vi "EnFlo_Lab_Temp_Control.vi"() -> ()   [LabVIEW 2010]
uses:
  ADAM Client/Sub VIs/ADAM Controls/Update_scan_value.ctl
panel:
  out "Total Delta Q":dbl
  out "Q output change from A Tunnel":dbl
  out "Desired Temp":dbl
  out "New Q":dbl
  out "Chiller water temp change OK?":bool
  out "Desired Chilled water temp":dbl
  out "Delta T Chiller":dbl
  out "Delta Q":dbl
  out "Temperature Error":dbl
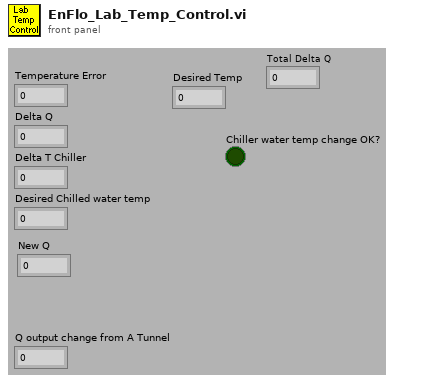
[diagram p1: front panel]
types:
  T1 = typedef "Update_scan_value.ctl" = cluster{"Channel Name":string, "New Value":dbl}
  T2 = enum16{"Append to Global", "Read Global then Clear"}
  T3 = typedef "Ch_description_ADAM.ctl" = cluster{"Ch Name":string, "Type":T4, "Function":T5, "Ch State":T6, "Calibration type":T7, "A":dbl, "B":dbl, "C":dbl, "D":dbl, "Comments":string, "Address":T8, "String":string, "Duty":u16}
  T4 = typedef "Module_type_ADAM.ctl" = enum16{"4011", "4012", "4013", "4014", "4016", "4017", "4018", "4021", "4050", "4052", "4053", "4060", "4080", "5000", "5017", "5018", "5024", "5051", "5056", "5060", "6060", "Tracker", "WEST", "GILL", "JEM", "VICI", "Vaisala", "DRUCK", "Run VI Named:", "IR2100", "PPT", "Comparator", "VIRTUAL", "Hold Value", "Read A", "Read Ch", "Coded", "Client Info", "Web Client", "X10", "Test"}
  T5 = typedef "Function_ADAM.ctl" = enum16{"Analogue Input", "Digital Input", "Event counter", "Event rate", "Analogue Output", "Digital Output", "Relay Output"}
  T6 = typedef "Channel_State.ctl" = enum16{"On", "Off", "Always On", "Always Off"}
  T7 = typedef "Calib_type_ADAM.ctl" = enum16{"Raw", "Bx + A", "Cx^2 + Bx + A", "Dx^3 + Cx^2 + Bx + A", "In Band", "Hi-Tec Q", "Hi-Tec M_dot", "Text"}
  T8 = typedef "Address.ctl" = cluster{"Main":i32, "Ch.":i32, "Sub":i32, "Port Name":string}
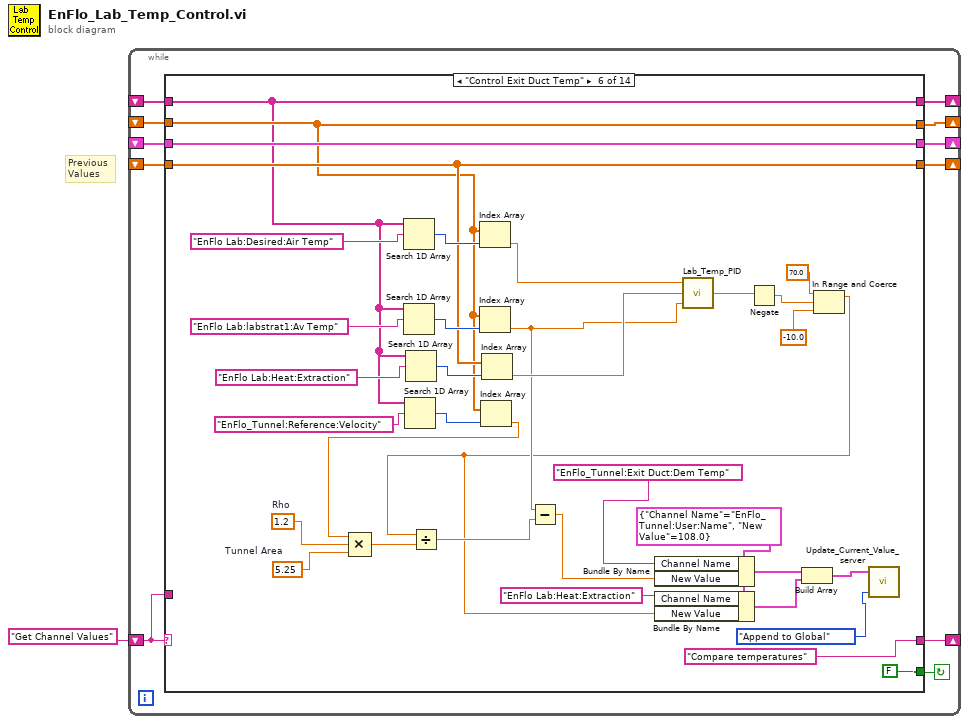
[diagram p0: block diagram]
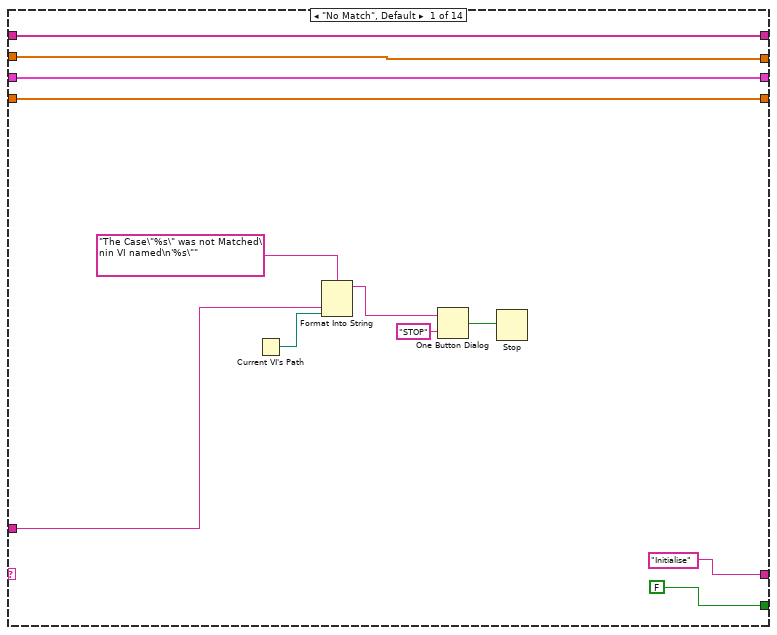
[diagram p2: hidden frame]
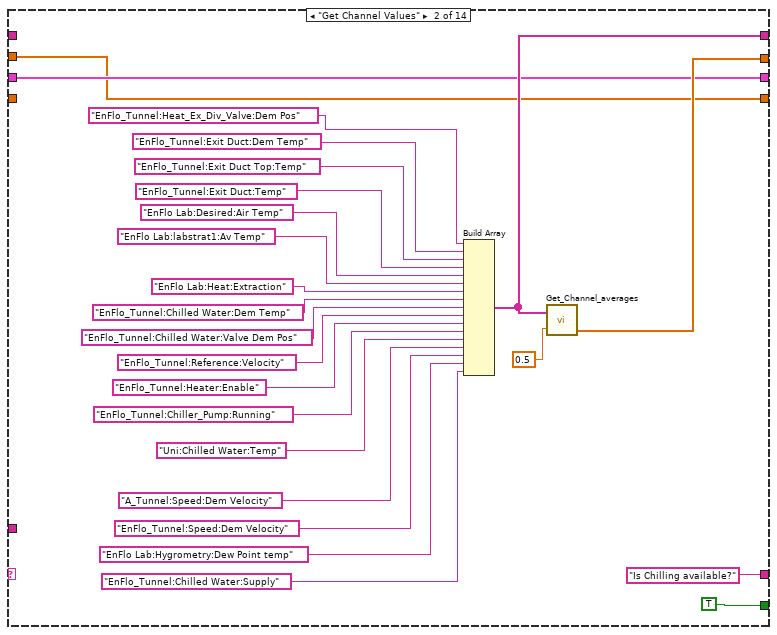
[diagram p3: hidden frame]
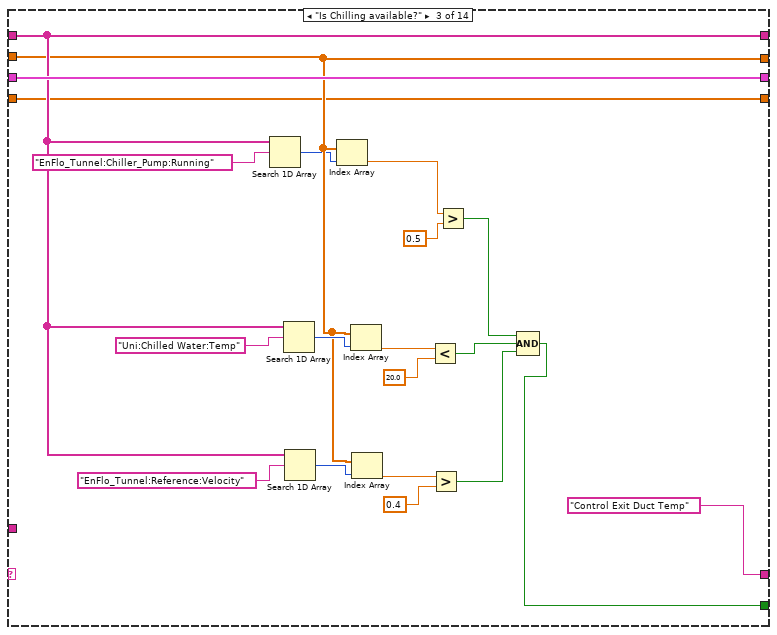
[diagram p4: hidden frame]
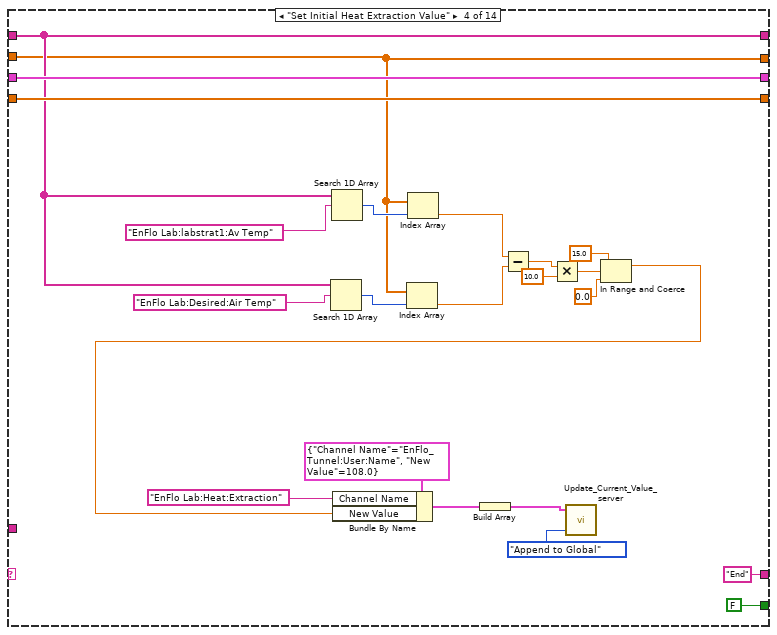
[diagram p5: hidden frame]
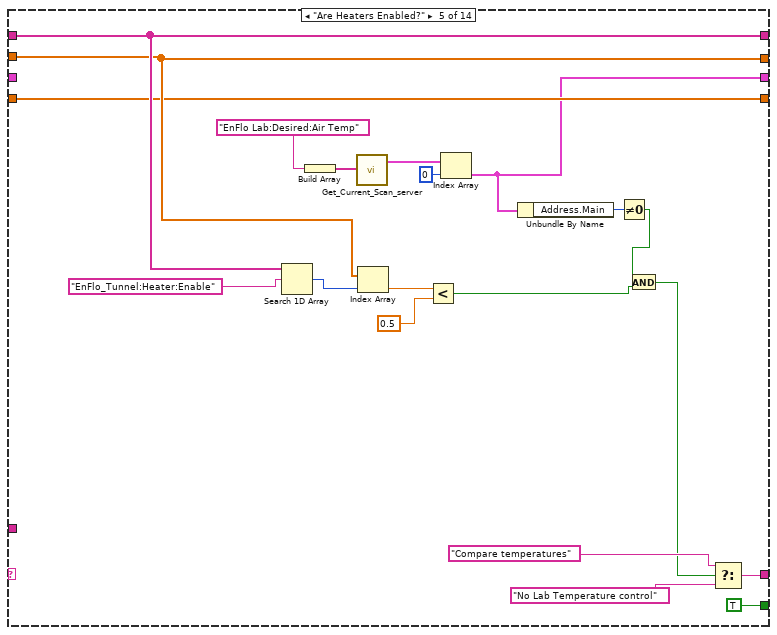
[diagram p6: hidden frame]
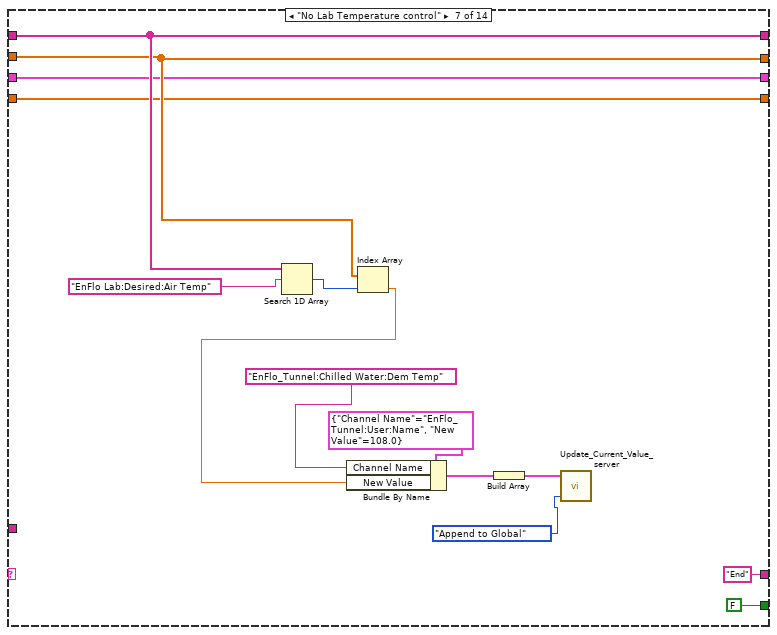
[diagram p7: hidden frame]
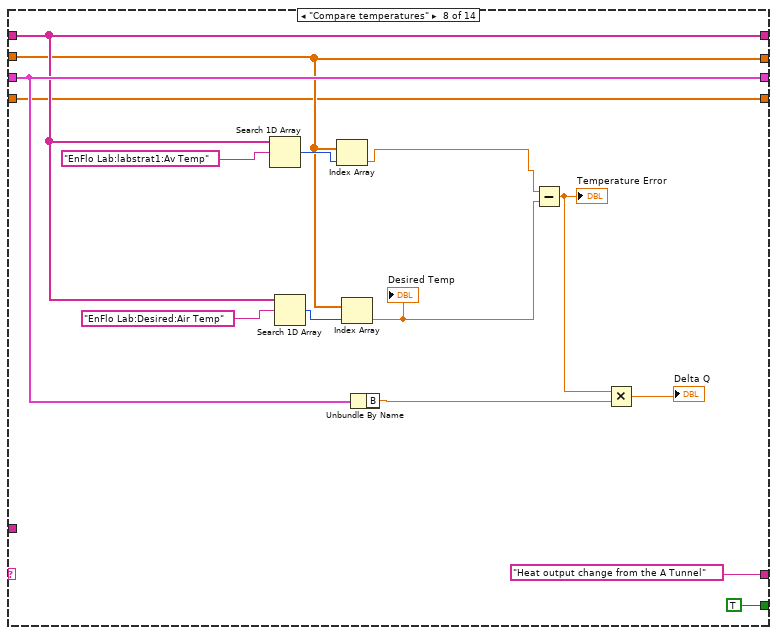
[diagram p8: hidden frame]
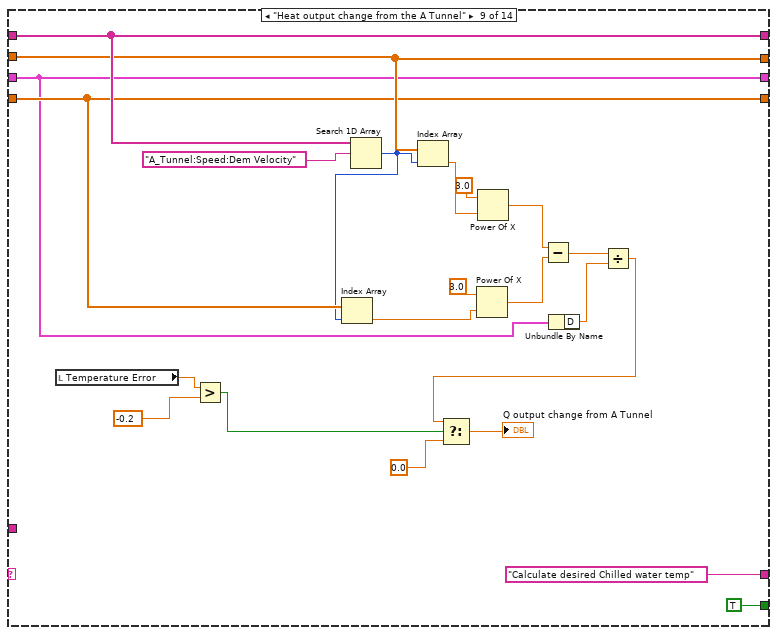
[diagram p9: hidden frame]
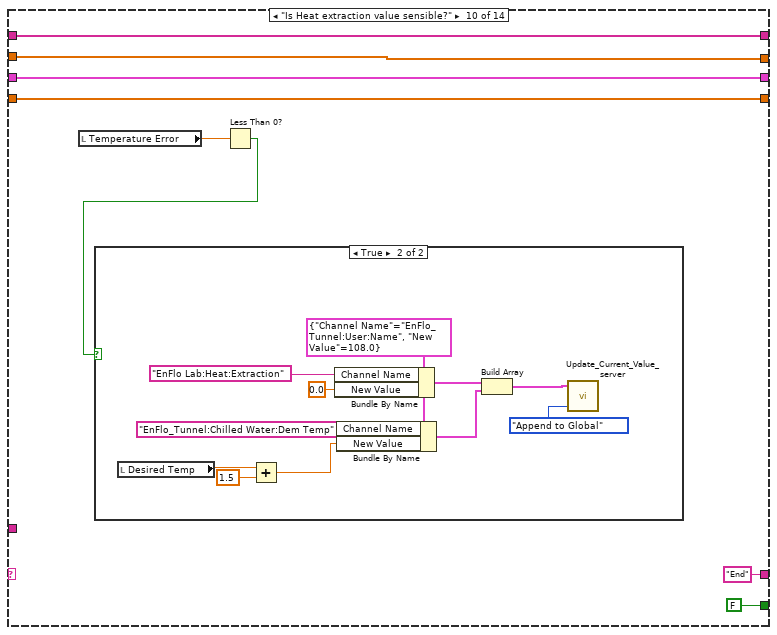
[diagram p10: hidden frame]
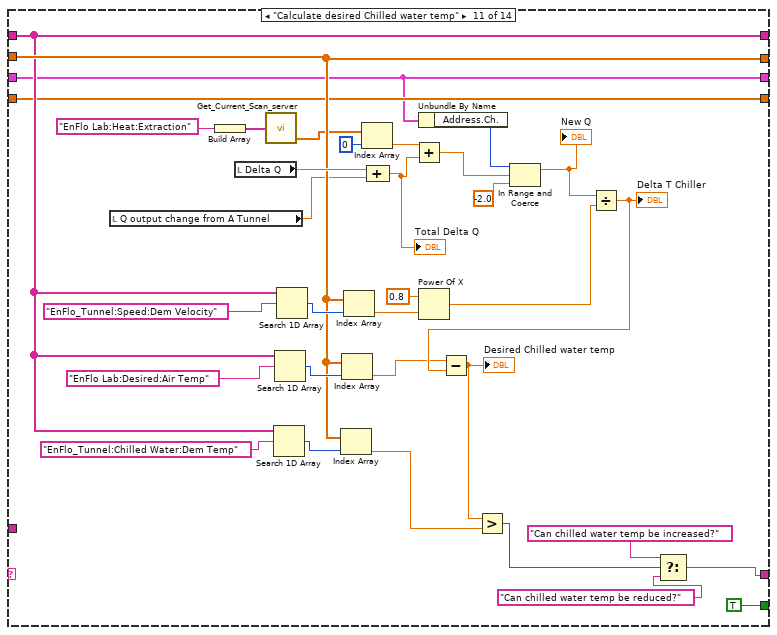
[diagram p12: hidden frame]
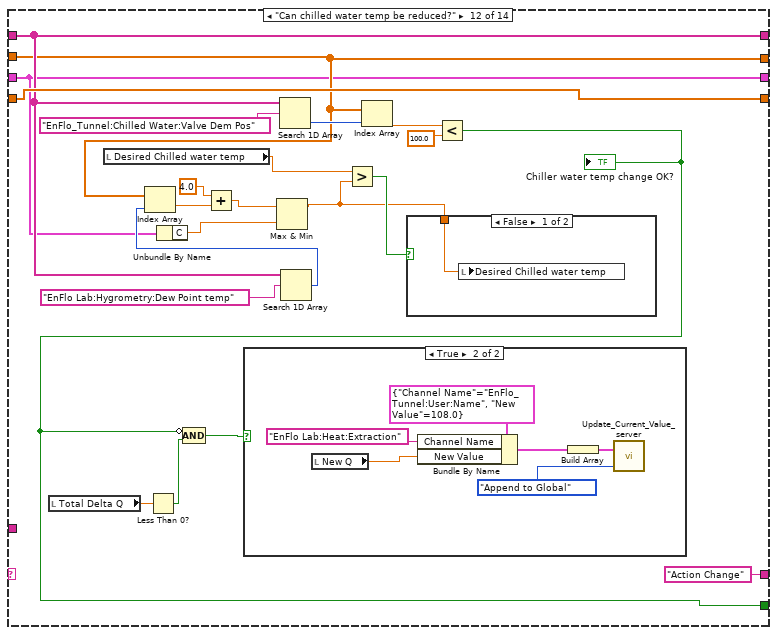
[diagram p13: hidden frame]
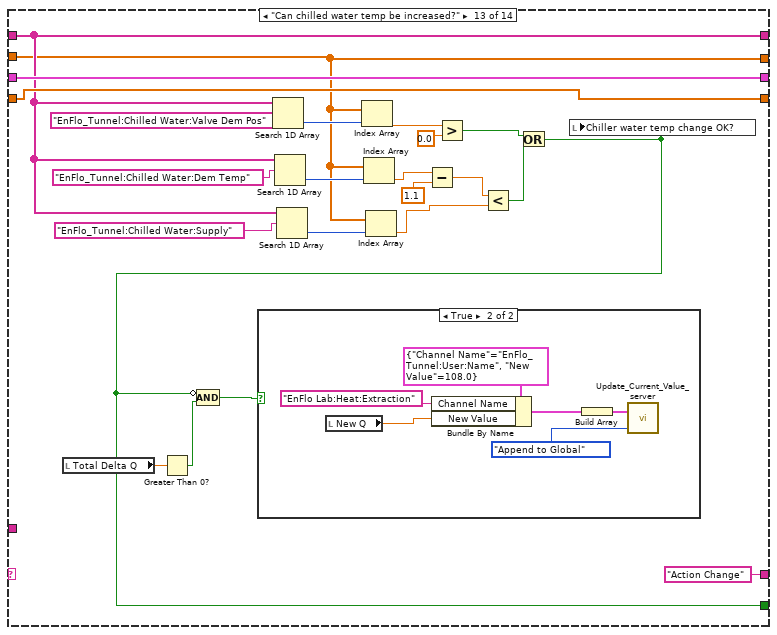
[diagram p16: hidden frame]
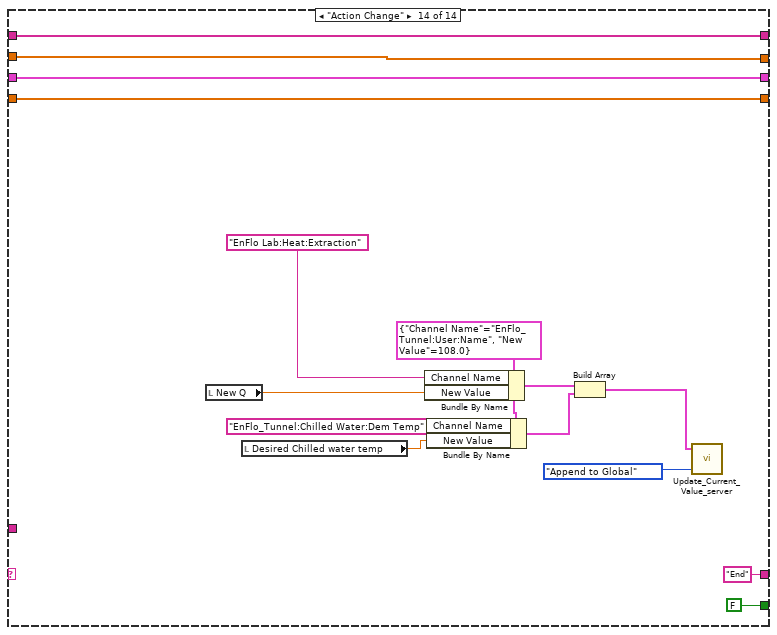
[diagram p18: hidden frame]
diagram:
  # "Previous\nValues"
  n1 = while {
    shift-left: "Get Channel Values" -> [w10]
    shift-right: [w11] -> _
    shift-right: [w8] -> _
    shift-left: _ -> [w6]
    shift-right: [w9] -> _
    shift-left: _ -> [w7]
    shift-right: [w5] -> _
    shift-left: _ -> [w4]
    shift-right: [w3] -> _
    shift-left: _ -> [w2]
    stop <- w12 continue-if-true
    n2 = case shown="\"Control Exit Duct Temp\"" w10 {
      tunnel: [FALSE TRUE w49 FALSE TRUE FALSE FALSE TRUE TRUE FALSE TRUE w262 w281 FALSE] -> w12
      tunnel: ["Initialise" "Is Chilling available?" "Control Exit Duct Temp" "End" ("f") w104 "Compare temperatures" "End" "Heat output change from the A Tunnel" "Calculate desired Chilled water temp" "End" ("f") w231 "Action Change" "Action Change" "End"] -> w11
      tunnel: w10 -> [w19 _ _ _ _ _ _ _ _ _ _ _ _ _]
      tunnel: [w16 w37 w55 w80 w109 w133 w157 w164 w195 w204 w238 w259 w291 w322] -> w9
      tunnel: [w15 w36 w56 w81 w110 w132 w158 w165 w196 w205 w237 w260 w292 w321] -> w8
      tunnel: w7 -> [w16 w32 w55 w80 w109 w133 w157 w164 w195 w204 w238 w259 w291 w322]
      tunnel: w6 -> [w15 _ w56 w81 w110 w132 w158 w165 w196 w205 w237 w260 w292 w321]
      tunnel: [w14 w34 w64 w92 w97 w144 w153 w173 w181 w206 w222 w257 w298 w320] -> w5
      tunnel: w4 -> [w14 w34 w64 w92 _ w144 w153 w173 w181 w206 w222 w257 w298 w320]
      tunnel: [w13 w32 w54 w89 w103 w134 w150 w163 w194 w199 w230 w267 w297 w313] -> w3
      tunnel: w2 -> [w13 _ w54 w89 w103 w134 w150 w163 w194 w199 w230 w267 w297 w313]
      frame "No Match", Default {
        n3 = Current VI's Path() -> (path=w18:path)
        n4 = Format Into String(format string="The Case\"%s\" was not Matched\nin VI named\n'%s\"" ("Format String"), w19, w18) -> (resulting string=w22:string)  [unwired: 2 in, 1 out]
        n5 = One Button Dialog(message=w22, button name ("OK")="STOP") -> (true=w20:bool)
        n6 = Stop(stop? (T)=w20) -> ()
      }
      frame "Get Channel Values" {
        n7 = Build Array("EnFlo_Tunnel:Heat_Ex_Div_Valve:Dem Pos", "EnFlo_Tunnel:Exit Duct:Dem Temp", "EnFlo_Tunnel:Exit Duct Top:Temp", "EnFlo_Tunnel:Exit Duct:Temp", "EnFlo Lab:Desired:Air Temp", "EnFlo Lab:labstrat1:Av Temp", "EnFlo Lab:Heat:Extraction", "EnFlo_Tunnel:Chilled Water:Dem Temp", "EnFlo_Tunnel:Chilled Water:Valve Dem Pos", "EnFlo_Tunnel:Reference:Velocity", "EnFlo_Tunnel:Heater:Enable", "EnFlo_Tunnel:Chiller_Pump:Running", "Uni:Chilled Water:Temp", "A_Tunnel:Speed:Dem Velocity", "EnFlo_Tunnel:Speed:Dem Velocity", "EnFlo Lab:Hygrometry:Dew Point temp", "EnFlo_Tunnel:Chilled Water:Supply") -> (w36:string[])
        n8 = call "Get_Channel_averages.vi"("Desired Ch Names"=w36, "Averaging time (mins)"=0.5) -> ("number"=w37:dbl[])  [unwired: 1 in, 2 out]
      }
      frame "Is Chilling available?" {
        n9 = Search 1D Array(1D array=w56, element="EnFlo_Tunnel:Chiller_Pump:Running") -> (index of element=w53:i32)  [unwired: 1 out]
        n10 = Search 1D Array(1D array=w56, element="Uni:Chilled Water:Temp") -> (index of element=w67:i32)  [unwired: 1 out]
        n11 = Search 1D Array(1D array=w56, element="EnFlo_Tunnel:Reference:Velocity") -> (index of element=w61:i32)  [unwired: 1 out]
        n12 = Index Array(array=w55, index=w53) -> (element=w50:dbl)
        n13 = Index Array(array=w55, index=w67) -> (element=w66:dbl)
        n14 = Index Array(array=w55, index=w61) -> (element=w62:dbl)
        n15 = Less?(x=w66, y=20.0) -> (x < y?=w59:bool)
        n16 = Greater?(x=w62, y=0.4) -> (0:w58:bool)
        n17 = Greater?(x=w50, y=0.5) -> (0:w51:bool)
        n18 = Compound Arithmetic op=AND(w51, w59, w58) -> (w49:bool)
      }
      frame "Set Initial Heat Extraction Value" {
        n19 = Search 1D Array(1D array=w81, element="EnFlo Lab:Desired:Air Temp") -> (index of element=w82:i32)  [unwired: 1 out]
        n20 = Search 1D Array(1D array=w81, element="EnFlo Lab:labstrat1:Av Temp") -> (index of element=w83:i32)  [unwired: 1 out]
        n21 = Index Array(array=w80, index=w82) -> (element=w77:dbl)
        n22 = Index Array(array=w80, index=w83) -> (element=w76:dbl)
        n23 = Subtract(x=w76, y=w77) -> (x-y=w75:dbl)
        n24 = Multiply(x=w75, y=10.0) -> (x*y=w73:dbl)
        n25 = In Range and Coerce(upper limit=15.0, x=w73, lower limit=0.0) -> (coerced(x)=w70:dbl)  [unwired: 1 out]
        n26 = Bundle By Name(cluster=T1 {"Channel Name"="EnFlo_Tunnel:User:Name", "New Value"=108.0} ("Update Scan Value Cluster"), "Channel Name"="EnFlo Lab:Heat:Extraction", "New Value"=w70) -> (w88:T1)
        n27 = Build Array(w88) -> (w85:T1[])
        n28 = call "Update_Current_Value_server.vi"("Mode"=T2."Append to Global", "Update array in"=w85) -> ()  [unwired: 1 in, 1 out]
      }
      frame "Are Heaters Enabled?" {
        n29 = Search 1D Array(1D array=w110, element="EnFlo_Tunnel:Heater:Enable") -> (index of element=w112:i32)  [unwired: 1 out]
        n30 = Build Array("EnFlo Lab:Desired:Air Temp") -> (w100:string[])
        n31 = call "Get_Current_Scan_server.vi"("Desired Channels"=w100) -> ("Ch Description Array"=w99:T3[])  [unwired: 2 out]
        n32 = Index Array(array=w109, index=w112) -> (element=w108:dbl)
        n33 = Less?(x=w108, y=0.5) -> (x < y?=w95:bool)
        n34 = Index Array(array=w99, index=0) -> (element=w97:T3)
        n35 = Unbundle By Name(w97) -> ("Address.Main"=w96:i32)
        n36 = Not Equal To 0?(x=w96) -> (x != 0?=w94:bool)
        n37 = And(x=w94, y=w95) -> (x .and. y?=w93:bool)
        n38 = Select(t="Compare temperatures", s=w93, f="No Lab Temperature control") -> (s? t:f=w104:string)
      }
      frame "Control Exit Duct Temp" {
        w113 = T1 {"Channel Name"="EnFlo_Tunnel:User:Name", "New Value"=108.0} ("Update Scan Value Cluster")
        w129 = 5.25  # Tunnel Area
        w130 = 1.2  # Rho
        n39 = Search 1D Array(1D array=w132, element="EnFlo Lab:Desired:Air Temp") -> (index of element=w147:i32)  [unwired: 1 out]
        n40 = Search 1D Array(1D array=w132, element="EnFlo Lab:labstrat1:Av Temp") -> (index of element=w142:i32)  [unwired: 1 out]
        n41 = Search 1D Array(1D array=w132, element="EnFlo_Tunnel:Reference:Velocity") -> (index of element=w135:i32)  [unwired: 1 out]
        n42 = Search 1D Array(1D array=w132, element="EnFlo Lab:Heat:Extraction") -> (index of element=w140:i32)  [unwired: 1 out]
        n43 = Index Array(array=w133, index=w147) -> (element=w141:dbl)
        n44 = Index Array(array=w133, index=w142) -> (element=w127:dbl)
        n45 = Index Array(array=w133, index=w135) -> (element=w131:dbl)
        n46 = Compound Arithmetic op=MULTIPLY(w131, w130, w129) -> (w128:dbl)
        n47 = Index Array(array=w134, index=w140) -> (element=w139:dbl)
        n48 = call "Lab_Temp_PID.vi"("Present Value"=w127, "Previous Control Sum"=w139, "Setpoint"=w141) -> ("Dem Output"=w121:dbl)
        n49 = Negate(x=w121) -> (-x=w120:dbl)
        n50 = In Range and Coerce(upper limit=70.0, x=w120, lower limit=-10.0) -> (coerced(x)=w115:dbl)  [unwired: 1 out]
        n51 = Divide(x=w115, y=w128) -> (x/y=w126:dbl)
        n52 = Subtract(x=w127, y=w126) -> (x-y=w122:dbl)
        n53 = Bundle By Name(cluster=w113, "Channel Name"="EnFlo_Tunnel:Exit Duct:Dem Temp", "New Value"=w122) -> (w117:T1)
        n54 = Bundle By Name(cluster=w113, "Channel Name"="EnFlo Lab:Heat:Extraction", "New Value"=w115) -> (w114:T1)
        n55 = Build Array(w117, w114) -> (w124:T1[])
        n56 = call "Update_Current_Value_server.vi"("Mode"=T2."Append to Global", "Update array in"=w124) -> ()  [unwired: 1 in, 1 out]
      }
      frame "No Lab Temperature control" {
        n57 = Search 1D Array(1D array=w158, element="EnFlo Lab:Desired:Air Temp") -> (index of element=w160:i32)  [unwired: 1 out]
        n58 = Index Array(array=w157, index=w160) -> (element=w151:dbl)
        n59 = Bundle By Name(cluster=T1 {"Channel Name"="EnFlo_Tunnel:User:Name", "New Value"=108.0} ("Update Scan Value Cluster"), "Channel Name"="EnFlo_Tunnel:Chilled Water:Dem Temp", "New Value"=w151) -> (w154:T1)
        n60 = Build Array(w154) -> (w149:T1[])
        n61 = call "Update_Current_Value_server.vi"("Mode"=T2."Append to Global", "Update array in"=w149) -> ()  [unwired: 1 in, 1 out]
      }
      frame "Compare temperatures" {
        n62 = Search 1D Array(1D array=w165, element="EnFlo Lab:labstrat1:Av Temp") -> (index of element=w176:i32)  [unwired: 1 out]
        n63 = Search 1D Array(1D array=w165, element="EnFlo Lab:Desired:Air Temp") -> (index of element=w175:i32)  [unwired: 1 out]
        n64 = Index Array(array=w164, index=w176) -> (element=w166:dbl)
        n65 = Index Array(array=w164, index=w175) -> (element=w167:dbl)
        "Desired Temp" <- w167
        n66 = Unbundle By Name(w173) -> ("B"=w172:dbl)
        n67 = Subtract(x=w166, y=w167) -> (x-y=w171:dbl)
        "Temperature Error" <- w171
        n68 = Multiply(x=w171, y=w172) -> (x*y=→"Delta Q":dbl)
      }
      frame "Heat output change from the A Tunnel" {
        n69 = local read "Temperature Error"() -> (w189:dbl)
        n70 = Greater?(x=w189, y=-0.2) -> (0:w187:bool)
        n71 = Search 1D Array(1D array=w196, element="A_Tunnel:Speed:Dem Velocity") -> (index of element=w193:i32)  [unwired: 1 out]
        n72 = Index Array(array=w194, index=w193) -> (element=w180:dbl)
        n73 = Index Array(array=w195, index=w193) -> (element=w179:dbl)
        n74 = Power Of X(1:w180, 2:3.0 ("x")) -> (0:w191:dbl)
        n75 = Power Of X(1:w179, 2:3.0 ("x")) -> (0:w192:dbl)
        n76 = Subtract(x=w192, y=w191) -> (x-y=w190:dbl)
        n77 = Unbundle By Name(w181) -> ("D"=w182:dbl)
        n78 = Divide(x=w190, y=w182) -> (x/y=w186:dbl)
        n79 = Select(t=w186, s=w187, f=0.0) -> (s? t:f=→"Q output change from A Tunnel":dbl)
      }
      frame "Is Heat extraction value sensible?" {
        n80 = local read "Temperature Error"() -> (w203:dbl)
        n81 = Less Than 0?(x=w203) -> (x < 0?=w202:bool)
        n82 = case shown="True" w202 {
          frame False {
          }
          frame True {
            w214 = T1 {"Channel Name"="EnFlo_Tunnel:User:Name", "New Value"=108.0} ("Update Scan Value Cluster")
            n83 = local read "Desired Temp"() -> (w211:dbl)
            n84 = Add(x=w211, y=1.5) -> (x+y=w209:dbl)
            n85 = Bundle By Name(cluster=w214, "Channel Name"="EnFlo Lab:Heat:Extraction", "New Value"=0.0) -> (w217:T1)
            n86 = Bundle By Name(cluster=w214, "Channel Name"="EnFlo_Tunnel:Chilled Water:Dem Temp", "New Value"=w209) -> (w213:T1)
            n87 = Build Array(w217, w213) -> (w208:T1[])
            n88 = call "Update_Current_Value_server.vi"("Mode"=T2."Append to Global", "Update array in"=w208) -> ()  [unwired: 1 in, 1 out]
          }
        }
      }
      frame "Calculate desired Chilled water temp" {
        n89 = local read "Q output change from A Tunnel"() -> (w229:dbl)
        n90 = Build Array("EnFlo Lab:Heat:Extraction") -> (w223:string[])
        n91 = local read "Delta Q"() -> (w248:dbl)
        n92 = call "Get_Current_Scan_server.vi"("Desired Channels"=w223) -> ("Numerical Values"=w225:dbl[])  [unwired: 2 out]
        n93 = Search 1D Array(1D array=w237, element="EnFlo_Tunnel:Chilled Water:Dem Temp") -> (index of element=w239:i32)  [unwired: 1 out]
        n94 = Search 1D Array(1D array=w237, element="EnFlo Lab:Desired:Air Temp") -> (index of element=w244:i32)  [unwired: 1 out]
        n95 = Search 1D Array(1D array=w237, element="EnFlo_Tunnel:Speed:Dem Velocity") -> (index of element=w250:i32)  [unwired: 1 out]
        n96 = Index Array(array=w238, index=w239) -> (element=w235:dbl)
        n97 = Index Array(array=w238, index=w244) -> (element=w241:dbl)
        n98 = Index Array(array=w238, index=w250) -> (element=w247:dbl)
        n99 = Index Array(array=w225, index=0) -> (element=w220:dbl)
        n100 = Compound Arithmetic op=ADD(w248, w229) -> (w219:dbl)
        "Total Delta Q" <- w219
        n101 = Add(x=w220, y=w219) -> (x+y=w218:dbl)
        n102 = Unbundle By Name(w222) -> ("Address.Ch."=w221:i32)
        n103 = Power Of X(1:w247, 2:0.8 ("y")) -> (0:w245:dbl)
        n104 = In Range and Coerce(upper limit=w221, x=w218, lower limit=-2.0) -> (coerced(x)=w227:dbl)  [unwired: 1 out]
        "New Q" <- w227
        n105 = Divide(x=w227, y=w245) -> (x/y=w242:dbl)
        "Delta T Chiller" <- w242
        n106 = Subtract(x=w241, y=w242) -> (x-y=w236:dbl)
        "Desired Chilled water temp" <- w236
        n107 = Greater?(x=w236, y=w235) -> (0:w234:bool)
        n108 = Select(t="Can chilled water temp be increased?", s=w234, f="Can chilled water temp be reduced?") -> (s? t:f=w231:string)
      }
      frame "Can chilled water temp be reduced?" {
        n109 = local read "Total Delta Q"() -> (w266:dbl)
        n110 = local read "Desired Chilled water temp"() -> (w268:dbl)
        n111 = Less Than 0?(x=w266) -> (x < 0?=w265:bool)
        n112 = Unbundle By Name(w257) -> ("C"=w256:dbl)
        n113 = Search 1D Array(1D array=w260, element="EnFlo_Tunnel:Chilled Water:Valve Dem Pos") -> (index of element=w273:i32)  [unwired: 1 out]
        n114 = Search 1D Array(1D array=w260, element="EnFlo Lab:Hygrometry:Dew Point temp") -> (index of element=w258:i32)  [unwired: 1 out]
        n115 = Index Array(array=w259, index=w258) -> (element=w254:dbl)
        n116 = Add(x=4.0, y=w254) -> (x+y=w252:dbl)
        n117 = Max & Min(x=w252, y=w256) -> (max(x,y)=w255:dbl)  [unwired: 1 out]
        n118 = Greater?(x=w268, y=w255) -> (0:w263:bool)
        n119 = Index Array(array=w259, index=w273) -> (element=w270:dbl)
        n120 = case shown="False" w263 {
          tunnel: w255 -> [w274 _]
          frame False {
            n121 = local write "Desired Chilled water temp"(w274) -> ()
          }
          frame True {
          }
        }
        n122 = Less?(x=w270, y=100.0) -> (x < y?=w262:bool)
        "Chiller water temp change OK?" <- w262
        n123 = Compound Arithmetic op=AND(invert w262, w265) -> (w264:bool)
        n124 = case shown="True" w264 {
          frame False {
          }
          frame True {
            n125 = local read "New Q"() -> (w277:dbl)
            n126 = Bundle By Name(cluster=T1 {"Channel Name"="EnFlo_Tunnel:User:Name", "New Value"=108.0} ("Update Scan Value Cluster"), "Channel Name"="EnFlo Lab:Heat:Extraction", "New Value"=w277) -> (w280:T1)
            n127 = Build Array(w280) -> (w275:T1[])
            n128 = call "Update_Current_Value_server.vi"("Mode"=T2."Append to Global", "Update array in"=w275) -> ()  [unwired: 1 in, 1 out]
          }
        }
      }
      frame "Can chilled water temp be increased?" {
        n129 = local read "Total Delta Q"() -> (w284:dbl)
        n130 = Greater Than 0?(x=w284) -> (x > 0?=w283:bool)
        n131 = Search 1D Array(1D array=w292, element="EnFlo_Tunnel:Chilled Water:Valve Dem Pos") -> (index of element=w303:i32)  [unwired: 1 out]
        n132 = Search 1D Array(1D array=w292, element="EnFlo_Tunnel:Chilled Water:Dem Temp") -> (index of element=w296:i32)  [unwired: 1 out]
        n133 = Search 1D Array(1D array=w292, element="EnFlo_Tunnel:Chilled Water:Supply") -> (index of element=w295:i32)  [unwired: 1 out]
        n134 = Index Array(array=w291, index=w303) -> (element=w300:dbl)
        n135 = Index Array(array=w291, index=w296) -> (element=w290:dbl)
        n136 = Index Array(array=w291, index=w295) -> (element=w287:dbl)
        n137 = Subtract(x=w290, y=1.1) -> (x-y=w288:dbl)
        n138 = Greater?(x=w300, y=0.0) -> (0:w285:bool)
        n139 = Less?(x=w288, y=w287) -> (x < y?=w286:bool)
        n140 = Or(x=w285, y=w286) -> (x .or. y?=w281:bool)
        n141 = Compound Arithmetic op=AND(invert w281, w283) -> (w282:bool)
        n142 = case shown="True" w282 {
          frame False {
          }
          frame True {
            n143 = local read "New Q"() -> (w306:dbl)
            n144 = Bundle By Name(cluster=T1 {"Channel Name"="EnFlo_Tunnel:User:Name", "New Value"=108.0} ("Update Scan Value Cluster"), "Channel Name"="EnFlo Lab:Heat:Extraction", "New Value"=w306) -> (w309:T1)
            n145 = Build Array(w309) -> (w304:T1[])
            n146 = call "Update_Current_Value_server.vi"("Mode"=T2."Append to Global", "Update array in"=w304) -> ()  [unwired: 1 in, 1 out]
          }
        }
        n147 = local write "Chiller water temp change OK?"(w281) -> ()
      }
      frame "Action Change" {
        w318 = T1 {"Channel Name"="EnFlo_Tunnel:User:Name", "New Value"=108.0} ("Update Scan Value Cluster")
        n148 = local read "New Q"() -> (w312:dbl)
        n149 = local read "Desired Chilled water temp"() -> (w315:dbl)
        n150 = Bundle By Name(cluster=w318, "Channel Name"="EnFlo Lab:Heat:Extraction", "New Value"=w312) -> (w319:T1)
        n151 = Bundle By Name(cluster=w318, "Channel Name"="EnFlo_Tunnel:Chilled Water:Dem Temp", "New Value"=w315) -> (w314:T1)
        n152 = Build Array(w319, w314) -> (w310:T1[])
        n153 = call "Update_Current_Value_server.vi"("Mode"=T2."Append to Global", "Update array in"=w310) -> ()  [unwired: 1 in, 1 out]
      }
    }
  }
